vi "Array_Size.vi"(9 "Array Size 2D":i8[][](array[numeric])=[[0, 4, 8], [1, 5, 9], [2, 6, 10], [3, 7, 11]], 10 "Array Size 1D":i8[](array[numeric])=[0, 1, 2, 3], 11 "Choose Array Size":T2) -> (1 "Size 2D":T1, 2 "Size 1D":i32)   [LabVIEW 2018]
uses:
  Controls/1D_2D.ctl
  Controls/Rows_Columns.ctl
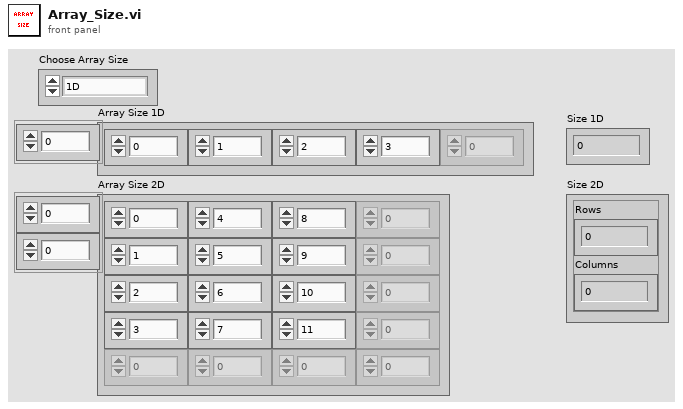
[diagram p1: front panel]
types:
  T1 = typedef "Rows_Columns.ctl" = cluster{"Rows":i32, "Columns":i32}
  T2 = typedef "1D_2D.ctl" = enum16{"1D", "2D"}
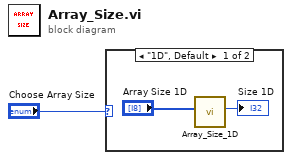
[diagram p0: block diagram]
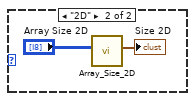
[diagram p2: hidden frame]
diagram:
  n1 = case shown="\"1D\", Default" "Choose Array Size" {
    frame "1D", Default {
      n2 = call "Array_Size_1D.vi"("Array"="Array Size 1D") -> ("Size"=→"Size 1D":i32)  [unwired: 10 in]
    }
    frame "2D" {
      n3 = call "Array_Size_2D.vi"("Array"="Array Size 2D") -> ("Size 2D"=→"Size 2D":T1)  [unwired: 10 in]
    }
  }
